vi "connect.vi"(8 "error in (no error)":errorcluster, 11 "TCPServer in":refnum<class "TCPServer.lvclass">) -> (0 "error out":errorcluster, 3 "TCPServer out":refnum<class "TCPServer.lvclass">)   [LabVIEW 2016, in "TCPServer.lvclass"]
uses:
  TCPServer.lvclass
  C:/Users/aanania/Documents/ts_monochromator_windows/ts_labview_tcp/TCPCommunicator/TCPCommunicator.lvclass
  TCPSettings/TCPSettings.lvclass/TCPSettings.ctl
  TCPCommunicator/TCPCommunicator.lvclass/TCPCommunicator.ctl
  TCPSettings/TCPSettings.lvclass
  TCPCommunicator/TCPCommunicator.lvclass
panel:
  out "port":u16
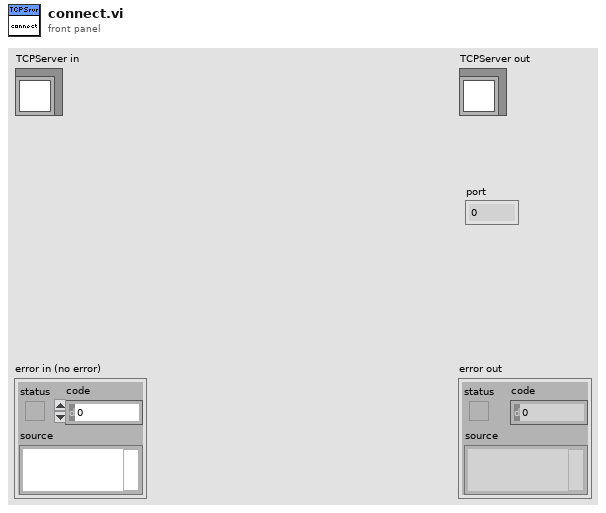
[diagram p1: front panel]
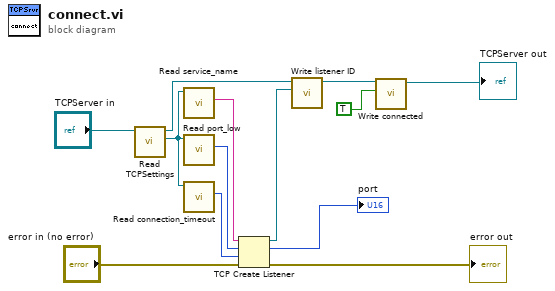
[diagram p0: block diagram]
diagram:
  n1 = call-dynamic "Read TCPSettings.vi"("TCPCommunicator in"="TCPServer in") -> ("TCPSettings.lvclass"=w10:refnum<class "TCPSettings.lvclass">, "TCPCommunicator out"=w2:refnum<class "TCPServer.lvclass">)  [unwired: 8 in, 1 out]
  n2 = call "Read service_name.vi"("TCPSettings in"=w10) -> ("service_name"=w12:string)  [unwired: 8 in, 2 out]
  n3 = call-dynamic "Read port_low.vi"("TCPSettings in"=w10) -> ("port_low"=w13:u16)  [unwired: 8 in, 2 out]
  n4 = call-dynamic "Read connection_timeout .vi"("TCPSettings in"=w10) -> ("connection_timeout"=w11:i32)  [unwired: 8 in, 2 out]
  n5 = TCP Create Listener(8:"error in (no error)", 9:w11, 10:w13, 11:w12) -> (0:→"error out":errorcluster, 2:→"port":u16, 3:w1:refnum<k5>)  [unwired: 1 out]
  n6 = call "Write listener ID.vi"("listener ID"=w1, "TCPCommunicator in"=w2) -> ("TCPCommunicator out"=w3:refnum<class "TCPServer.lvclass">)  [unwired: 8 in, 1 out]
  n7 = call "Write connected.vi"("connected"=TRUE, "TCPCommunicator in"=w3) -> ("TCPCommunicator out"=→"TCPServer out":refnum<class "TCPServer.lvclass">)  [unwired: 8 in, 1 out]
